vi "Interval.vi"(8 "error in (no error)":errorcluster, 11 "DiscoveryService in":refnum<class "DiscoveryService.lvclass">) -> (0 "error out":errorcluster, 2 "Interval S":dbl, 3 "DiscoveryService out":refnum<class "DiscoveryService.lvclass">)   [LabVIEW 2020, in "Vecto.lvlib" / "DiscoveryService.lvclass"]
uses:
  DiscoveryService.lvclass
  DiscoveryService.lvclass/DiscoveryService.ctl
  Node Config/Node Config.lvclass
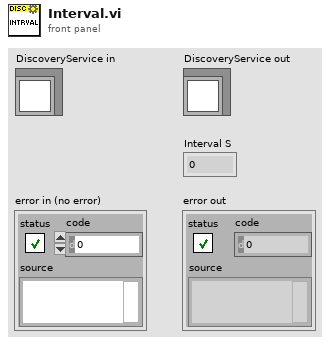
[diagram p1: front panel]
types:
  T1 = typedef "Vecto.lvlib/Discovery Info.ctl" = cluster{"Address":string, "Port":u16, "Interval S":dbl}
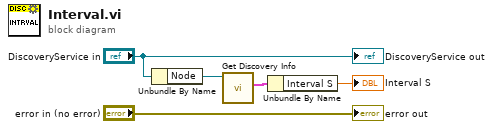
[diagram p0: block diagram]
diagram:
  n1 = Unbundle By Name("DiscoveryService in") -> ("Node"=w5:refnum<class "Node Config.lvclass">)
  n2 = call "Get Discovery Info.vi"("Node in"=w5) -> ("Discovery Info"=w4:T1)  [unwired: 8 in, 2 out]
  n3 = Unbundle By Name(w4) -> ("Interval S"=→"Interval S":dbl)
  "error out" <- "error in (no error)"
  "DiscoveryService out" <- "DiscoveryService in"
